vi "CAENHV Get Sys Prop List.vi"(8 "error in (no error)":errorcluster, 11 "handle":i32) -> (0 "error out":errorcluster, 2 "PropNameList":string[](array[string]), 3 "NumProp":u16)   [LabVIEW 2009, in "CAENHVWrapper.lvlib"]
doc: "CAENHVLIB_API CAENHVRESULT CAENHV_GetSysPropList(int handle, \n ushort *NumProp, char **PropNameList);"
uses:
  <userlib>/CAENHVWrapper/CAENHVWrapper.lvlib
  <vilib>/Utility/importsl/GetValueByPointer/GetValueByPointer.xnode
  <vilib>/Utility/importsl/GetValueByPointer/datatype.ctl
  <userlib>/CAENHVWrapper/CAENHVWrapper.dll
  resource/lvimptsl.dll
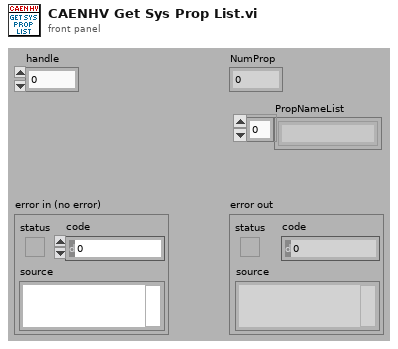
[diagram p1: front panel]
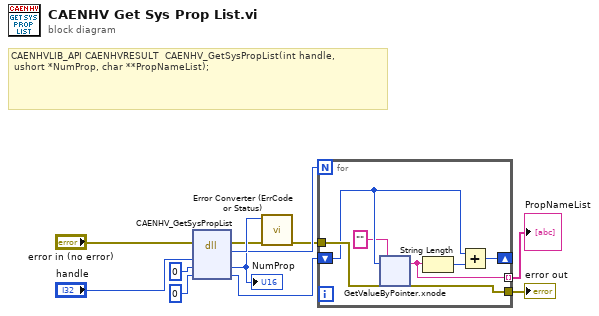
[diagram p0: block diagram]
diagram:
  # "CAENHVLIB_API CAENHVRESULT  CAENHV_GetSysPropList(int handle, \n ushort *NumProp, char **PropNameList);"
  n1 = dll-call lib="C:/Program Files/National Instruments/LabVIEW 2009/user.lib/CAENHVWrapper/CAENHVWrapper.*" fn="CAENHV_GetSysPropList"(error in="error in (no error)", "handle"="handle", "NumProp"=u16 0, "PropNameList"=i64 0) -> (error out=w7:errorcluster, "return type"=w8:i32, "NumProp"=w5:u16, "PropNameList"=w3:i64)  [unwired: 3 in, 1 out]
  "NumProp" <- w5
  n2 = call <userlib>:"Error Converter (ErrCode or Status).vi"("error in (no error)"=w7, "error code"=w8) -> ("error out"=w4:errorcluster)  [unwired: 9 in]
  n3 = for {
    N: w5 -> [_]
    shift-right: [w14] -> _
    shift-left: w3 -> [w16]
    tunnel: w4 -> [w18]
    tunnel: [w17] -> w1
    tunnel: [w12] -> w2 mode=indexing
    n4 = xnode "GetValueByPointer.xnode"("Pointer"=w16, "InputType"="", "ErrorIn"=w18) -> ("Output"=w12:string, "ErrorOut"=w17:errorcluster)  [unwired: 1 in]
    n5 = String Length(string=w12) -> (length=w15:i32)
    n6 = Add(x=w16, y=w15) -> (x+y=w14:i64)
  }
  "error out" <- w1
  "PropNameList" <- w2
